vi "Array - Failure Message.vi"() -> ()   [LabVIEW 2017, in "Transparent Assertions.Tests.lvlib" / "Assert Collection Empty.lvlib"]
uses:
  Assert Collection Empty.lvlib
  src/Transparent Assertions/Transparent Assertions.lvlib
panel:
  out "error out":errorcluster
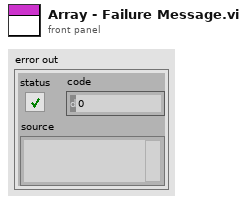
[diagram p1: front panel]
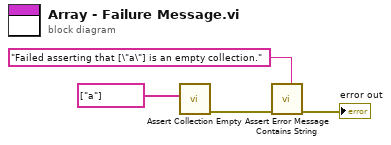
[diagram p0: block diagram]
diagram:
  n1 = call "Assert Collection Empty.vi"("Collection"=string[] ["a"]) -> ("error out"=w3:errorcluster)  [unwired: 10 in]
  n2 = call "Assert Error Message Contains String.vi"("Expected"="Failed asserting that [\"a\"] is an empty collection.", "error in (no error)"=w3) -> ("error out"=→"error out":errorcluster)  [unwired: 9 in]
